vi "retrieveCalibratedData.vi"(8 "error in (no error)":errorcluster, 11 "TEI9150 in":refnum<class "Tovey9150.lvclass">) -> (0 "error out":errorcluster, 3 "TEI9150 out":refnum<class "Tovey9150.lvclass">)   [LabVIEW 2015]
uses:
  <vilib>/regexp/Match Regular Expression.xnode
  Tovey9150.lvclass
  <userlib>/Common/SerialProtocols/SerialCommunicator/SerialCommunicator.lvclass
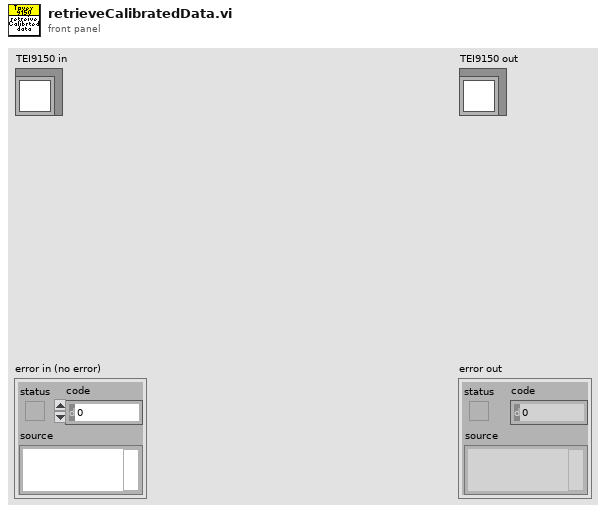
[diagram p1: front panel]
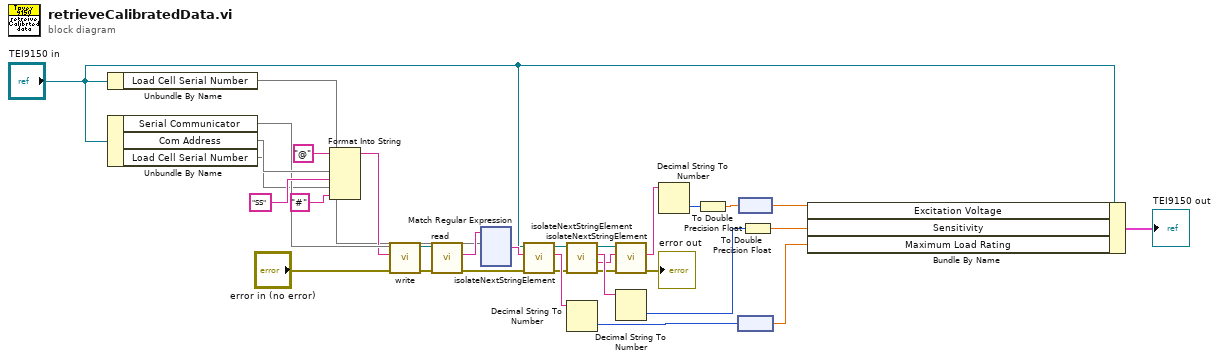
[diagram p0: block diagram]
diagram:
  n1 = Unbundle By Name("TEI9150 in") -> ("Load Cell Serial Number"=w21)
  n2 = Unbundle By Name("TEI9150 in") -> ("Serial Communicator"=w28, "Com Address"=w32, "Load Cell Serial Number"=w24)
  n3 = Format Into String(initial string="@", w32, "SS" ("input 2"), w24, "#" ("input 4")) -> (resulting string=w26:string)  [unwired: 2 in, 1 out]
  n4 = call-dynamic "write.vi"("error in (no error)"="error in (no error)", "writeString"=w26, "SerialCommunicator in"=w28) -> ("error out"=w29:errorcluster, "SerialCommunicator out"=w30:refnum<class "SerialCommunicator.lvclass">)  [unwired: 7 in]
  n5 = call-dynamic "read.vi"("error in (no error)"=w29, "SerialCommunicator in"=w30) -> ("error out"=w10:errorcluster, "stringRead"=w22:string)  [unwired: 7 in, 1 out]
  n6 = xnode "Match Regular Expression"("input string"=w22, "regular expression"=w21) -> ("after match"=w20:string)  [unwired: 4 in, 4 out]
  n7 = call "isolateNextStringElement.vi"("error in (no error)"=w10, "inputString"=w20, "TEI9150 in"="TEI9150 in") -> ("error out"=w9:errorcluster, "extractedSegment"=w16:string, "TEI9150 out"=w19:refnum<class "Tovey9150.lvclass">)  [unwired: 5 in, 1 out]
  n8 = call "isolateNextStringElement.vi"("error in (no error)"=w9, "TEI9150 in"=w19) -> ("error out"=w8:errorcluster, "remainingString"=w7:string, "extractedSegment"=w13:string, "TEI9150 out"=w18:refnum<class "Tovey9150.lvclass">)  [unwired: 6 in]
  n9 = Decimal String To Number(string=w16) -> (number=w15:i32)  [unwired: 2 in, 1 out]
  n10 = call "isolateNextStringElement.vi"("error in (no error)"=w8, "inputString"=w7, "TEI9150 in"=w18) -> ("error out"=→"error out":errorcluster, "extractedSegment"=w6:string)  [unwired: 5 in, 2 out]
  n11 = Decimal String To Number(string=w13) -> (number=w12:i32)  [unwired: 2 in, 1 out]
  n12 = Decimal String To Number(string=w6) -> (number=w5:i32)  [unwired: 2 in, 1 out]
  n13 = To Double Precision Float(number=w5) -> (double precision float=w4:dbl)
  n14 = node(w15) -> (w14:dbl[unit])
  n15 = node(w4) -> (w3:dbl[unit])
  n16 = To Double Precision Float(number=w12) -> (double precision float=w11:dbl)
  n17 = Bundle By Name(cluster="TEI9150 in", "Excitation Voltage"=w3, "Sensitivity"=w11, "Maximum Load Rating"=w14) -> (→"TEI9150 out":cluster{})
